vi "Poll.vi"(8 "error in (no error)":errorcluster, 10 "Lamp.lvclass":refnum<class "Lamp.lvclass">, 11 "Button in":refnum<class "Button.lvclass">) -> (0 "error out":errorcluster, 2 "Lamp out":refnum<class "Lamp.lvclass">, 3 "Button out":refnum<class "Button.lvclass">)   [LabVIEW 2018, in "Button.lvclass"]
uses:
  Button.lvclass
  Lamp/Lamp.lvclass
  Button.lvclass/Button.ctl
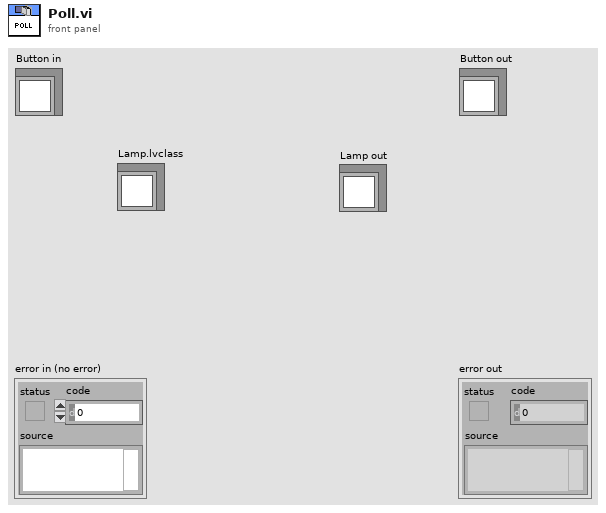
[diagram p1: front panel]
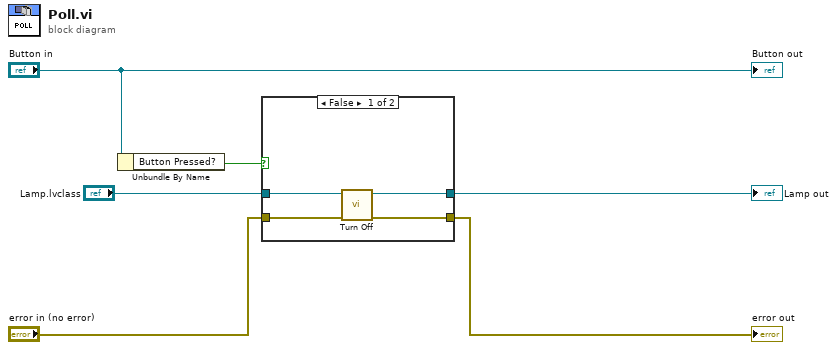
[diagram p0: block diagram]
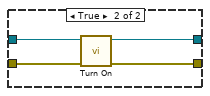
[diagram p2: hidden frame]
diagram:
  n1 = Unbundle By Name("Button in") -> ("Button Pressed?"=w5:bool)
  n2 = case shown="False" w5 {
    tunnel: "Lamp.lvclass" -> [w10 w13]
    tunnel: "error in (no error)" -> [w9 w14]
    tunnel: [w8 w12] -> w2
    tunnel: [w7 w11] -> w1
    frame False {
      n3 = call-dynamic "Turn Off.vi"("error in (no error)"=w9, "Lamp in"=w10) -> ("error out"=w8:errorcluster, "Lamp out"=w7:refnum<class "Lamp.lvclass">)  [unwired: 8 in]
    }
    frame True {
      n4 = call-dynamic "Turn On.vi"("error in (no error)"=w14, "Lamp in"=w13) -> ("error out"=w12:errorcluster, "Lamp out"=w11:refnum<class "Lamp.lvclass">)  [unwired: 8 in]
    }
  }
  "error out" <- w2
  "Lamp out" <- w1
  "Button out" <- "Button in"
